vi "experiment.vi"() -> ()   [LabVIEW 2014]
uses:
  <instrlib>/niDMM/nidmm.llb/niDMM Waveform Function.ctl
  <instrlib>/niDMM/nidmm.llb/niDMM Read Waveform (waveform data).vi
  <vilib>/DAQmx/create/channels.llb/DAQmx Create Channel (AO-Voltage-Basic).vi
  <vilib>/DAQmx/configure/timing.llb/DAQmx Timing (Sample Clock).vi
  <vilib>/measure/maresamp.llb/Resample Waveform (single shot).vi
  <vilib>/ptbypt/Frequency Domain.llb/Real FFT PtByPt.vi
  <vilib>/DAQmx/write.llb/DAQmx Write (Analog Wfm 1Chan NSamp).vi
  <vilib>/measure/NI_MAPro.lvlib
  <vilib>/measure/NI_MABase.lvlib
  <resource>/objmgr/daqmx.rc
  <vilib>/ptbypt/NI_PtbyPt.lvlib
panel:
  out "frequency 2":dbl
  out "x-y":dbl
  in  "error in":errorcluster caption="错误输入"
  out "frequency":dbl
  out "df":dbl
  out "输出簇":cluster{"f0":dbl, "df":dbl, "magnitude":dbl[]}(graph)
  out "Actual Number":i32
  out "元素":waveform(dbl)[](graph)
  in  "停止":bool
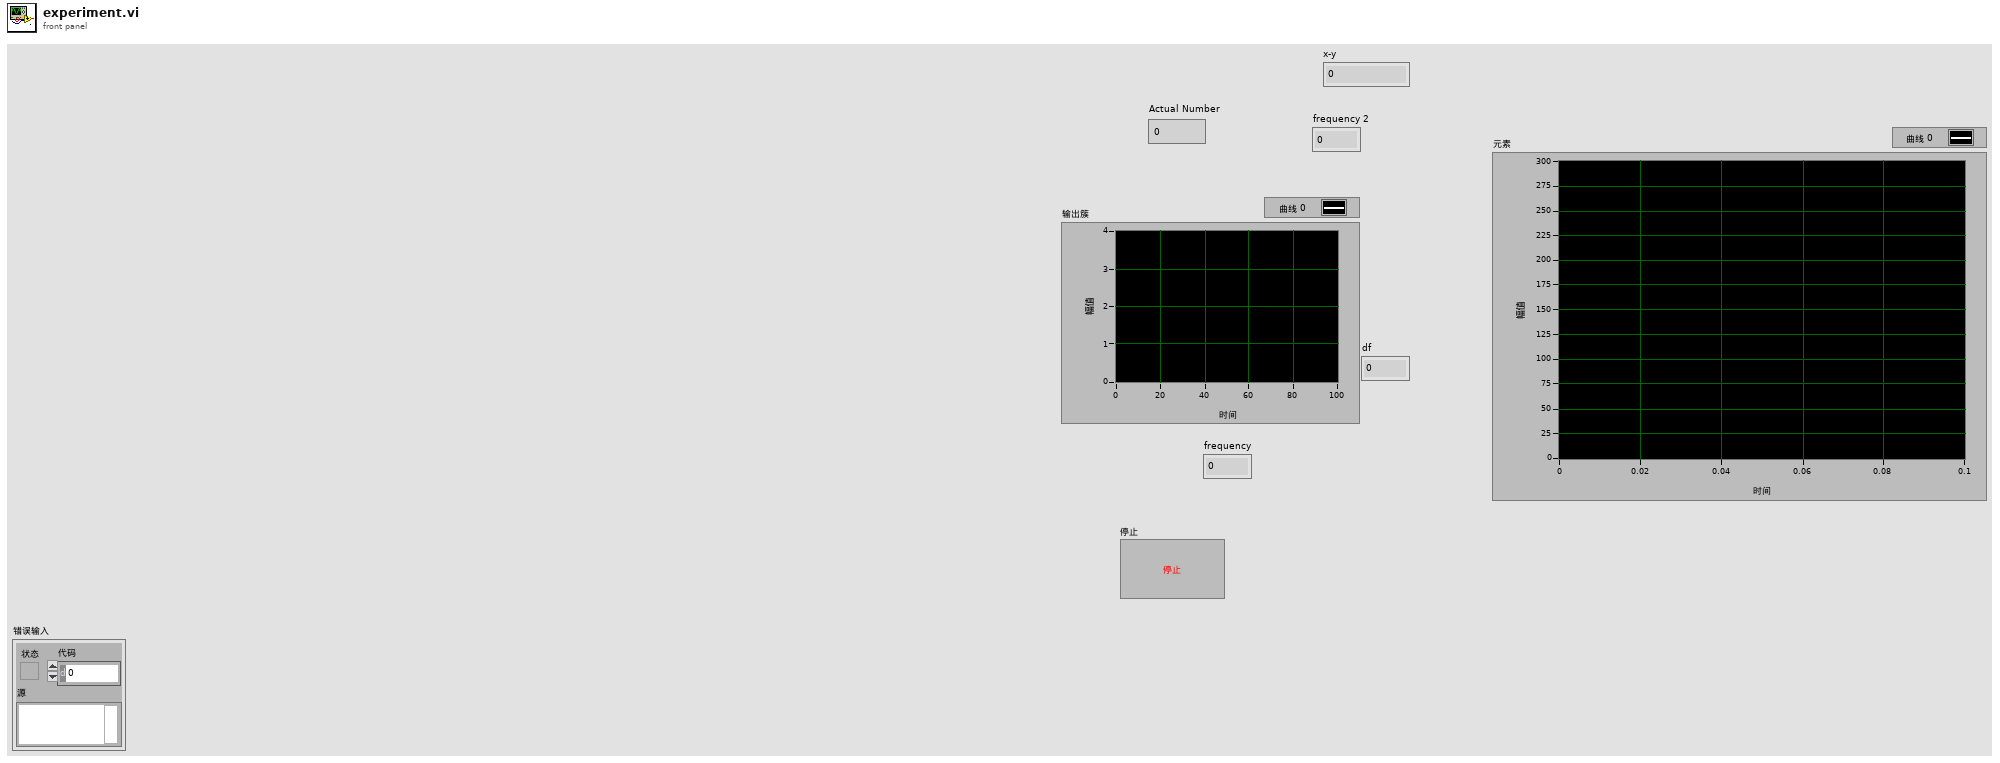
[diagram p1: front panel]
types:
  T1 = typedef "niDMM Waveform Function.ctl" = i32
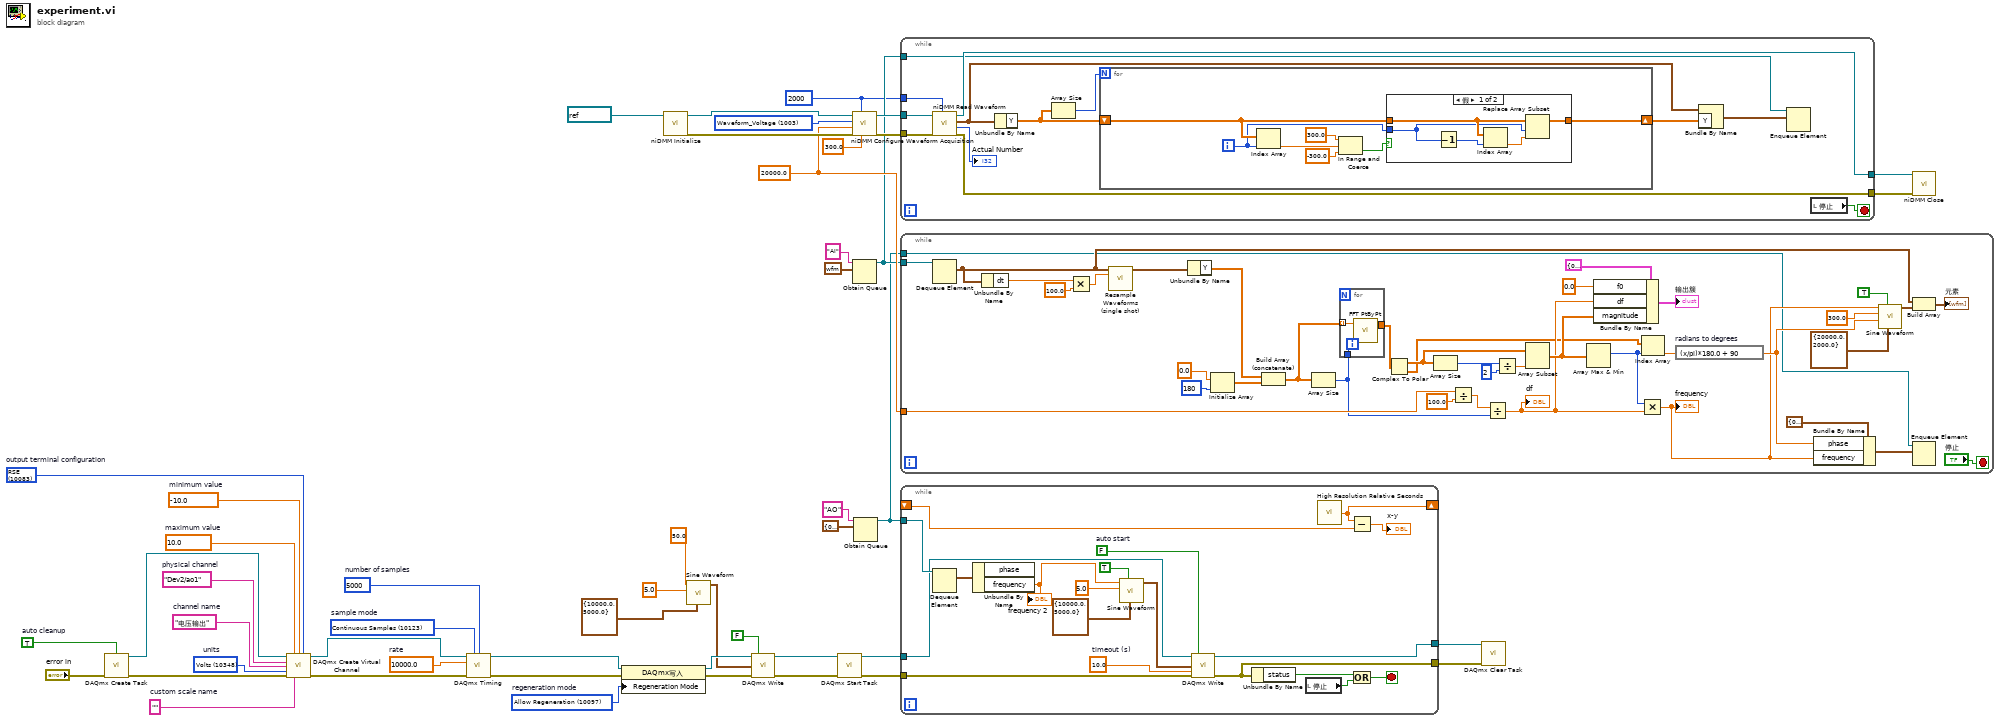
[diagram p0: block diagram]
diagram:
  w17 = 10097 items=["Allow Regeneration"=10097, "Do Not Allow Regeneration"=10158]  # regeneration mode
  w19 = 10123 items=["Finite Samples"=10178, "Continuous Samples"=10123, "Hardware Timed Single Point"=12522]  # sample mode
  w20 = 5000  # number of samples
  w21 = 10000.0  # rate
  w24 = 10083 items=["Default"=-1, "RSE"=10083, "Differential"=10106, "Pseudodifferential"=12529]  # output terminal configuration
  w25 = 10348 items=["Volts"=10348, "From Custom Scale"=10065]  # units
  w26 = "电压输出"  # channel name
  w28 = ""  # custom scale name
  w29 = -10.0  # minimum value
  w30 = 10.0  # maximum value
  w31 = "Dev2/ao1"  # physical channel
  w33 = TRUE  # auto cleanup
  w36 = 2000 ("Waveform Points")
  w44 = 20000.0 ("Rate")
  w49 = T1 1003 items=["Waveform_Voltage"=1003, "Waveform_Current"=1004] ("Function")
  n1 = call <vilib>:"DAQmx Create Task.vi"("auto cleanup"=w33, "error in"="error in") -> ("task out"=w32:refnum<k21>, "error out"=w34:errorcluster)  [unwired: 12 in]
  n2 = call-poly <vilib>:"DAQmx Create Virtual Channel.vi"("task in"=w32, "maximum value"=w30, "minimum value"=w29, "output terminal configuration"=w24, "physical channels"=w31, "name to assign"=w26, "units"=w25, "error in"=w34, "custom scale name"=w28) -> ("task out"=w22:refnum<k21>, "error out"=w27:errorcluster)  [unwired: 5 in]
  n3 = call-poly <vilib>:"DAQmx Timing.vi"("task/channels in"=w22, "sample mode"=w19, "samples per channel"=w20, "rate"=w21, "error in"=w27) -> ("task out"=w18:refnum<k21>, "error out"=w23:errorcluster)  [unwired: 9 in]
  n4 = property class="DAQmx写入"(reference=w18, error in=w23, "Regeneration Mode"=w17) -> (reference out=w9:refnum<k21>, error out=w7:errorcluster)
  n5 = call <instrlib>:"niDMM Initialize.vi"("Instrument Descriptor"=refnum<k15> "Dev1" ("instrument handle")) -> ("error out"=w46:errorcluster, "instrument handle out"=w47:refnum<k15>)  [unwired: 9 in]
  n6 = call <vilib>:"Sine Waveform.vi"("sampling info"=cluster{"Fs":dbl, "#s":dbl} {"Fs"=10000.0, "#s"=5000.0}, "amplitude"=5.0, "frequency"=50.0) -> ("signal out"=w4:waveform(dbl))  [unwired: 7 in, 1 out]
  n7 = call-poly <vilib>:"DAQmx Write.vi"("task/channels in"=w9, "auto start"=FALSE, "data"=w4, "error in"=w7) -> ("task out"=w8:refnum<k21>, "error out"=w6:errorcluster)  [unwired: 9 in, 1 out]
  n8 = call <vilib>:"DAQmx Start Task.vi"("task/channels in"=w8, "error in"=w6) -> ("task out"=w13:refnum<k21>, "error out"=w12:errorcluster)  [unwired: 12 in]
  n9 = call <instrlib>:"niDMM Configure Waveform Acquisition.vi"("Range"=300.0, "Waveform Points"=w36, "error in (no error)"=w46, "Rate"=w44, "Function"=w49, "instrument handle"=w47) -> ("error out"=w41:errorcluster, "instrument handle out"=w42:refnum<k15>)  [unwired: 4 in]
  n10 = Obtain Queue(name (unnamed)="AI" ("名称（未命名）"), element data type=waveform(dbl) {"t0"=timestamp(0 s since 1904-01-01), "dt"=0.0, "Y"=[]} ("Waveform Data")) -> (queue out=w38:refnum<queue>)  [unwired: 3 in, 2 out]
  n11 = Obtain Queue(name (unnamed)="AO" ("名称（未命名）"), element data type=cluster{"phase":dbl, "frequency":dbl} {"phase"=0.0, "frequency"=0.0}) -> (queue out=w14:refnum<queue>)  [unwired: 3 in, 2 out]
  n12 = while {
    tunnel: w42 -> [w62]
    tunnel: w41 -> [w61]
    tunnel: [w60] -> w40
    tunnel: [w59] -> w39
    tunnel: w38 -> [w58]
    tunnel: w36 -> [w56]
    stop <- w57 stop-if-true
    n13 = call-poly <instrlib>:"niDMM Read Waveform.vi"("Number To Read"=w56, "error in (no error)"=w61, "instrument handle"=w62) -> ("error out"=w59:errorcluster, "Actual Number"=→"Actual Number":i32, "Waveform Data"=w54:waveform(dbl), "instrument handle out"=w60:refnum<k15>)  [unwired: 5 in]
    n14 = Unbundle By Name(w54) -> ("Y"=w51:dbl[])
    n15 = Array Size(array=w51) -> (size(s)=w50:i32)
    n16 = for {
      N: w50 -> [_]
      shift-right: [w69] -> w53
      shift-left: w51 -> [w65]
      i -> [w63]
      n17 = Index Array(array=w65, index=w63) -> (element=w64:dbl)
      n18 = In Range and Coerce(upper limit=300.0 ("上限"), x=w64, lower limit=-300.0 ("下限")) -> (In Range?=w66:bool)  [unwired: 1 out]
      n19 = case shown="假" w66 {
        tunnel: w65 -> [w73 w75]
        tunnel: [w72 w75] -> w69
        tunnel: w63 -> [w71 _]
        frame False {
          n20 = Decrement(x=w71) -> (x-1=w74:i32)
          n21 = Index Array(array=w73, index=w74) -> (element=w70:dbl)
          n22 = Replace Array Subset(array=w73, new element=w70, index=w71) -> (w72:dbl[])
        }
        frame True {
        }
      }
    }
    n23 = Bundle By Name(cluster=w54, "Y"=w53) -> (w52:waveform(dbl))
    n24 = Enqueue Element(queue=w58, element=w52) -> ()  [unwired: 2 in, 3 out]
    n25 = local read "停止"() -> (w57:bool)
  }
  n26 = while {
    tunnel: w44 -> [w103]
    tunnel: w38 -> [w113]
    tunnel: w14 -> [w80]
    stop <- "停止" stop-if-true
    n27 = Dequeue Element(queue=w113) -> (element=w89:waveform(dbl))  [unwired: 2 in, 3 out]
    n28 = Unbundle By Name(w89) -> ("dt"=w101:dbl)
    n29 = Multiply(x=w101, y=100.0) -> (x*y=w99:dbl)
    n30 = call-poly <vilib>:"Resample Waveforms (single shot).vi"("waveform in"=w89, "dt"=w99) -> ("resampled waveform out"=w88:waveform(dbl))  [unwired: 10 in, 3 out]
    n31 = Unbundle By Name(w88) -> ("Y"=w112:dbl[])
    n32 = Initialize Array(0.0 ("元素"), 180 ("维数大小")) -> (w105:dbl[])
    n33 = Build Array (concatenate)(w112, w105) -> (w77:dbl[])
    n34 = Array Size(array=w77) -> (size(s)=w78:i32)
    n35 = for {
      tunnel: w78 -> [w117]
      tunnel: w77 -> [w116] mode=indexing
      tunnel: [w115] -> w76
      n36 = call-poly <vilib>:"FFT PtByPt.vi"("sample length"=w117, "x"=w116) -> ("FFT{X}"=w115:cdb[])  [unwired: 2 in, 1 out]
    }
    n37 = Complex To Polar(r * e^(i*theta)=w76) -> (r=w109:dbl[], theta=w86:dbl[])
    n38 = Array Size(array=w109) -> (size(s)=w94:i32)
    n39 = Divide(x=w103, y=100.0) -> (x/y=w104:dbl)
    n40 = Divide(x=w104, y=w78) -> (x/y=w96:dbl)
    "df" <- w96
    n41 = Divide(x=w94, y=2) -> (x/y=w93:dbl)
    n42 = Array Subset(array=w109, length=w93) -> (w97:dbl[])  [unwired: 1 in]
    n43 = Array Max & Min(array=w97) -> (max index (indices)=w85:i32)  [unwired: 3 out]
    n44 = Bundle By Name(cluster=cluster{"f0":dbl, "df":dbl, "magnitude":dbl[]} {"f0"=0.0, "df"=0.0, "magnitude"=[]} ("magnitude"), "f0"=0.0, "df"=w96, "magnitude"=w97) -> (→"输出簇":cluster{"f0":dbl, "df":dbl, "magnitude":dbl[]})
    n45 = Multiply(x=w85, y=w96) -> (x*y=w81:dbl)
    "frequency" <- w81
    n46 = Index Array(array=w86, index=w85) -> (element=w84:dbl)
    n47 = expression code="(x/pi)*180.0 + 90" "radians to degrees"(w84) -> (w82:dbl)
    n48 = Bundle By Name(cluster=cluster{"phase":dbl, "frequency":dbl} {"phase"=0.0, "frequency"=0.0}, "phase"=w82, "frequency"=w81) -> (w79:cluster{"phase":dbl, "frequency":dbl})
    n49 = call <vilib>:"Sine Waveform.vi"("sampling info"=cluster{"Fs":dbl, "#s":dbl} {"Fs"=20000.0, "#s"=2000.0}, "reset signal"=TRUE, "phase"=w82, "amplitude"=300.0, "frequency"=w81) -> ("signal out"=w91:waveform(dbl))  [unwired: 5 in, 1 out]
    n50 = Build Array(w89, w91) -> (→"元素":waveform(dbl)[])
    n51 = Enqueue Element(queue=w80, element=w79) -> ()  [unwired: 2 in, 3 out]
  }
  n52 = while {
    tunnel: w13 -> [w128]
    tunnel: w12 -> [w127]
    tunnel: w14 -> [w134]
    tunnel: [w122] -> w11
    tunnel: [w121] -> w10
    shift-right: [w118] -> _
    shift-left: _ -> [w119]
    stop <- w125 stop-if-true
    w135 = 10.0  # timeout (s)
    w136 = FALSE  # auto start
    n53 = Dequeue Element(queue=w134) -> (element=w133:cluster{"phase":dbl, "frequency":dbl})  [unwired: 2 in, 3 out]
    n54 = Unbundle By Name(w133) -> ("frequency"=w132:dbl)  [unwired: 1 out]
    "frequency 2" <- w132
    n55 = call <vilib>:"Sine Waveform.vi"("sampling info"=cluster{"Fs":dbl, "#s":dbl} {"Fs"=10000.0, "#s"=5000.0}, "reset signal"=TRUE, "amplitude"=5.0, "frequency"=w132) -> ("signal out"=w129:waveform(dbl))  [unwired: 6 in, 1 out]
    n56 = call-poly <vilib>:"DAQmx Write.vi"("task/channels in"=w128, "auto start"=w136, "data"=w129, "timeout"=w135, "error in"=w127) -> ("task out"=w122:refnum<k21>, "error out"=w121:errorcluster)  [unwired: 8 in, 1 out]
    n57 = Unbundle By Name(w121) -> ("status"=w126:bool)
    n58 = local read "停止"() -> (w124:bool)
    n59 = call <vilib>:"High Resolution Relative Seconds.vi"() -> ("relative seconds"=w118:dbl)
    n60 = Subtract(x=w118, y=w119) -> (x-y=→"x-y":dbl)
    n61 = Or(x=w126, y=w124) -> (x .or. y?=w125:bool)
  }
  n62 = call <vilib>:"DAQmx Clear Task.vi"("task in"=w11, "error in"=w10) -> ()  [unwired: 13 in, 1 out]
  n63 = call <instrlib>:"niDMM Close.vi"("error in (no error)"=w39, "instrument handle"=w40) -> ()  [unwired: 9 in, 1 out]
